vi "RT-FPGA函数重置.vi"(4 "9213转换时间":enum8{"High Speed", "High Resolution"}(ring), 5 "9205AI Channel Settings":T4(array[cluster])=[{"Voltage Range"=enum."+/- 10V", "Terminal Mode"=enum."RSE"}, {"Voltage Range"=enum."+/- 10V", "Terminal Mode"=enum."RSE"}, {"Voltage Range"=enum."+/- 10V", "Terminal Mode"=enum."RSE"}, {"Voltage Range"=enum."+/- 10V", "Terminal Mode"=enum."RSE"}, {"Voltage Range"=enum."+/- 10V", "Terminal Mode"=enum."RSE"}, {"Voltage Range"=enum."+/- 10V", "Terminal Mode"=enum."RSE"}, {"Voltage Range"=enum."+/- 10V", "Terminal Mode"=enum."RSE"}, {"Voltage Range"=enum."+/- 10V", "Terminal Mode"=enum."RSE"}, {"Voltage Range"=enum."+/- 10V", "Terminal Mode"=enum."RSE"}, {"Voltage Range"=enum."+/- 10V", "Terminal Mode"=enum."RSE"}, {"Voltage Range"=enum."+/- 10V", "Terminal Mode"=enum."RSE"}, {"Voltage Range"=enum."+/- 10V", "Terminal Mode"=enum."RSE"}, {"Voltage Range"=enum."+/- 10V", "Terminal Mode"=enum."RSE"}, {"Voltage Range"=enum."+/- 10V", "Terminal Mode"=enum."RSE"}, {"Voltage Range"=enum."+/- 10V", "Terminal Mode"=enum."RSE"}, {"Voltage Range"=enum."+/- 10V", "Terminal Mode"=enum."RSE"}, {"Voltage Range"=enum."+/- 10V", "Terminal Mode"=enum."RSE"}, {"Voltage Range"=enum."+/- 10V", "Terminal Mode"=enum."RSE"}, {"Voltage Range"=enum."+/- 10V", "Terminal Mode"=enum."RSE"}, {"Voltage Range"=enum."+/- 10V", "Terminal Mode"=enum."RSE"}, {"Voltage Range"=enum."+/- 10V", "Terminal Mode"=enum."RSE"}, {"Voltage Range"=enum."+/- 10V", "Terminal Mode"=enum."RSE"}, {"Voltage Range"=enum."+/- 10V", "Terminal Mode"=enum."RSE"}, {"Voltage Range"=enum."+/- 10V", "Terminal Mode"=enum."RSE"}, {"Voltage Range"=enum."+/- 10V", "Terminal Mode"=enum."RSE"}], 6 "update9213":bool=TRUE, 7 "9205Update AI Setings":bool, 8 "错误输入":errorcluster, 9 "9229采样率":T1=1 items=["", "50.000 kS/s (NI 9229)", "25.000 kS/s (NI 9229)", "16.667 kS/s (NI 9229)", "12.500 kS/s (NI 9229)", "10.000 kS/s (NI 9229)", "8.333 kS/s (NI 9229)", "7.143 kS/s (NI 9229)", "6.250 kS/s (NI 9229)", "5.556 kS/s (NI 9229)", "5.000 kS/s (NI 9229)", "4.545 kS/s (NI 9229)", "4.167 kS/s (NI 9229)", "3.846 kS/s (NI 9229)", "3.571 kS/s (NI 9229)", "3.333 kS/s (NI 9229)", "3.125 kS/s (NI 9229)", "2.941 kS/s (NI 9229)", "2.778 kS/s (NI 9229)", "2.632 kS/s (NI 9229)", "2.500 kS/s (NI 9229)", "2.381 kS/s (NI 9229)", "2.273 kS/s (NI 9229)", "2.174 kS/s (NI 9229)", "2.083 kS/s (NI 9229)", "2.000 kS/s (NI 9229)", "1.923 kS/s (NI 9229)", "1.852 kS/s (NI 9229)", "1.786 kS/s (NI 9229)", "1.724 kS/s (NI 9229)", "1.667 kS/s (NI 9229)", "1.613 kS/s (NI 9229)"], 10 "9205Count(uSec)":u32=1000) -> (0 "错误输出":errorcluster, 3 "FPGA VI引用输出":refnum<k20>)   [LabVIEW 2013]
uses:
  <vilib>/LabVIEW Targets/FPGA/cRIO/shared/nicrio_ModuleControls/nicrio_cRIO-9205_VoltageRange.ctl
  <vilib>/LabVIEW Targets/FPGA/cRIO/shared/nicrio_ModuleControls/nicrio_cRIO-9205_TerminalMode.ctl
  <vilib>/LabVIEW Targets/FPGA/cRIO/shared/nicrio_ModuleControls/nicrio_cRIO-9229_DataRatesRing.ctl
  <vilib>/FPGAPlugInAG/Dynamic/niLvFpga_Reset_Dynamic.vi
  <vilib>/rvi/interface/common/niFpgaWaitOnOcc.vi
  <vilib>/Utility/error.llb/Error Cluster From Error Code.vi
  <vilib>/rvi/errors/niLvFpgaAdjustHostInterfaceError.vi
  <vilib>/FPGAPlugInAG/Dynamic/niLvFpga_Run_Dynamic.vi
  <vilib>/rvi/interface/nirviMethod/nirviMethod.xnode
  <vilib>/rvi/interface/nirviReadWriteControl/nirviReadWriteControl.xnode
  NiFpgaLv.dll
  <vilib>/rvi/interface/Simulation/niFpgaSimulationCallBeginRW.vi
  <vilib>/FPGAPlugInAG/Dynamic/niLvFpga_ConfigureFifo_Dynamic.vi
  <vilib>/rvi/errors/niLvFpgaMergeErrorWithErrorCode.vi
  <vilib>/FPGAPlugInAG/Dynamic/niLvFpga_ReadFifo_Dynamic.vi
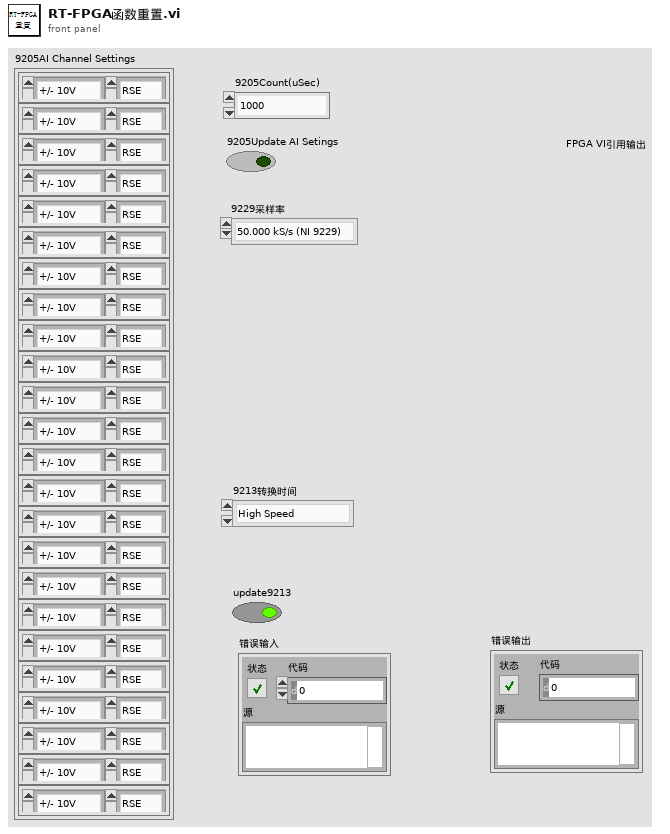
[diagram p1: front panel]
types:
  T1 = typedef "nicrio_cRIO-9229_DataRatesRing.ctl" = u8
  T2 = typedef "nicrio_cRIO-9205_VoltageRange.ctl" = enum8{"+/- 10V", "+/- 5V", "+/- 1V", "+/- 200mV"}
  T3 = typedef "nicrio_cRIO-9205_TerminalMode.ctl" = enum8{"RSE", "NRSE", "DIFF"}
  T4 = cluster{"Voltage Range":T2, "Terminal Mode":T3}[]
  T5 = cluster{i32, "Voltage Range":T2, "Terminal Mode":T3}
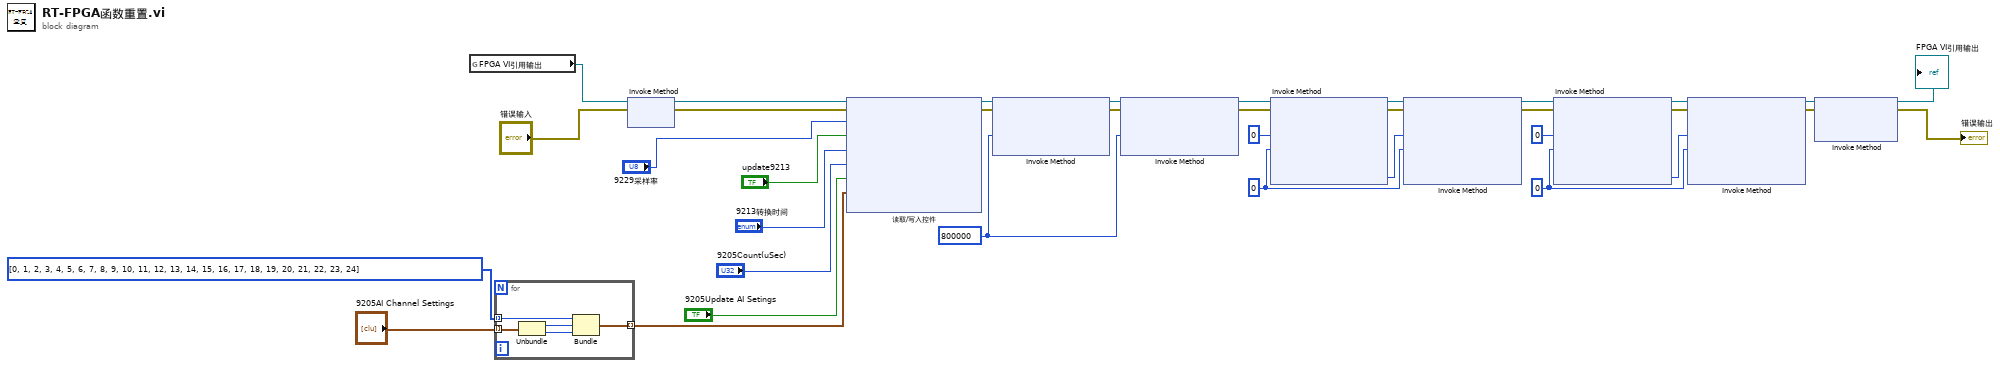
[diagram p0: block diagram]
diagram:
  w12 = 0 ("超时(ms)")
  w18 = 0 ("超时(ms)")
  w24 = u32 800000 ("请求的深度")
  n1 = global read "RT-FPGA引用全局.vi" "FPGA VI引用输出"() -> (w2:refnum<k20>)
  n2 = for {
    tunnel: "9205AI Channel Settings" -> [w40] mode=indexing
    tunnel: i32[] [0, 1, 2, 3, 4, 5, 6, 7, 8, 9, 10, 11, 12, 13, 14, 15, 16, 17, 18, 19, 20, 21, 22, 23, 24] -> [w39] mode=indexing
    tunnel: [w36] -> w29 mode=indexing
    n3 = Unbundle(w40) -> ("Voltage Range"=w38:T2, "Terminal Mode"=w37:T3)
    n4 = Bundle(w39, "Voltage Range"=w38, "Terminal Mode"=w37) -> (w36:T5)  [unwired: 1 in]
  }
  n5 = xnode "Invoke Method"("FPGA VI引用输入"=w2, "错误输入"="错误输入") -> ("FPGA VI引用输出"=w35:refnum<k20>, "错误输出"=w34:errorcluster)
  n6 = xnode "读取/写入控件"("FPGA VI引用输入"=w35, "错误输入"=w34, "9229采样率"="9229采样率", "update9213"="update9213", "9213转换时间"="9213转换时间", "9205Count(uSec)"="9205Count(uSec)", "9205Update AI Setings"="9205Update AI Setings", "9205AI DEFINE"=w29) -> ("FPGA VI引用输出"=w26:refnum<k20>, "错误输出"=w25:errorcluster)  [unwired: 1 in]
  n7 = xnode "Invoke Method"("FPGA VI引用输入"=w26, "错误输入"=w25, "请求的深度"=w24) -> ("FPGA VI引用输出"=w9:refnum<k20>, "错误输出"=w8:errorcluster)  [unwired: 1 out]
  n8 = xnode "Invoke Method"("FPGA VI引用输入"=w9, "错误输入"=w8, "请求的深度"=w24) -> ("FPGA VI引用输出"=w23:refnum<k20>, "错误输出"=w22:errorcluster)  [unwired: 1 out]
  n9 = xnode "Invoke Method"("FPGA VI引用输入"=w23, "错误输入"=w22, "元素数量"=u32 0, "超时(ms)"=w18) -> ("FPGA VI引用输出"=w21:refnum<k20>, "错误输出"=w20:errorcluster, "剩余元素"=w17:u32)  [unwired: 1 out]
  n10 = xnode "Invoke Method"("FPGA VI引用输入"=w21, "错误输入"=w20, "元素数量"=w17, "超时(ms)"=w18) -> ("FPGA VI引用输出"=w7:refnum<k20>, "错误输出"=w6:errorcluster)  [unwired: 2 out]
  n11 = xnode "Invoke Method"("FPGA VI引用输入"=w7, "错误输入"=w6, "元素数量"=u32 0, "超时(ms)"=w12) -> ("FPGA VI引用输出"=w16:refnum<k20>, "错误输出"=w15:errorcluster, "剩余元素"=w14:u32)  [unwired: 1 out]
  n12 = xnode "Invoke Method"("FPGA VI引用输入"=w16, "错误输入"=w15, "元素数量"=w14, "超时(ms)"=w12) -> ("FPGA VI引用输出"=w11:refnum<k20>, "错误输出"=w10:errorcluster)  [unwired: 2 out]
  n13 = xnode "Invoke Method"("FPGA VI引用输入"=w11, "错误输入"=w10) -> ("FPGA VI引用输出"=→"FPGA VI引用输出":refnum<k20>, "错误输出"=→"错误输出":errorcluster)  [unwired: 1 in]
